vi "GA Get Di Reverse Count.vi"(7 "nCount":i16, 8 "error in (no error)":errorcluster caption="错误输入（无错误）", 9 "pReverseCount":u32, 10 "diIndex":i16, 11 "nDiType":i16) -> (0 "error out":errorcluster caption="错误输出", 1 "pReverseCount out":u32, 3 "function return":i32)   [LabVIEW 2015, in "GAS.lvlib"]
doc: "extern \"C\" __declspec(dllimport) int GA_GetDiReverseCount(short nDiType,short diIndex,unsigned long *pReverseCount,short nCount=1);"
uses:
  <userlib>/BP_GAS/GAS.lvlib
  <userlib>/BP_GAS/GAS.dll
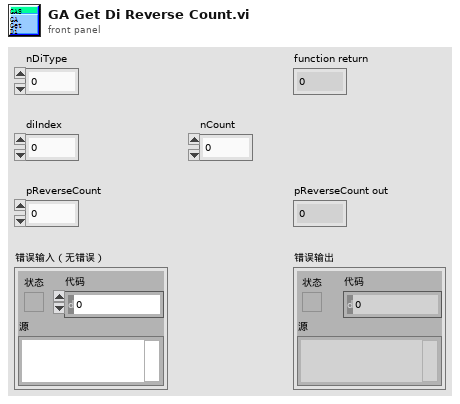
[diagram p1: front panel]
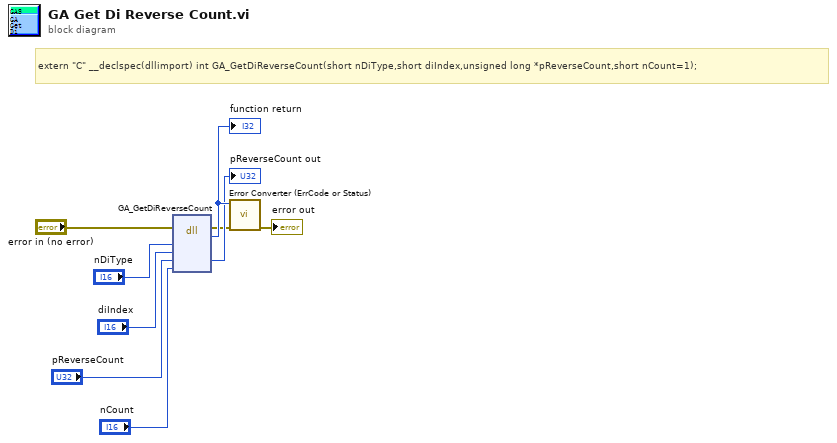
[diagram p0: block diagram]
diagram:
  # "extern \"C\" __declspec(dllimport) int GA_GetDiReverseCount(short nDiType,short diIndex,unsigned long *pReverseCount,short nCount=1);"
  n1 = dll-call lib="E:/Program Files (x86)/National Instruments/LabVIEW 2015/user.lib/BP_GAS/GAS.*" fn="GA_GetDiReverseCount"(error in="error in (no error)", "nDiType"="nDiType", "diIndex"="diIndex", "pReverseCount"="pReverseCount", "nCount"="nCount") -> (error out=w2:errorcluster, w9:i32, "pReverseCount"=→"pReverseCount out":u32)  [unwired: 5 in, 1 out]
  "function return" <- w9
  n2 = call "Error Converter (ErrCode or Status).vi"("error in (no error)"=w2, "error code"=w9) -> ("error out"=→"error out":errorcluster)  [unwired: 9 in]
